vi "Create.vi"(8 "error in (no error)":errorcluster, 10 "Data File":path) -> (0 "error out":errorcluster, 3 "Account Database out":refnum<class "Account Database.lvclass">)   [LabVIEW 2020, in "Account Database.lvclass"]
uses:
  Account Database.lvclass
  Account Database.lvclass/Account Database.ctl
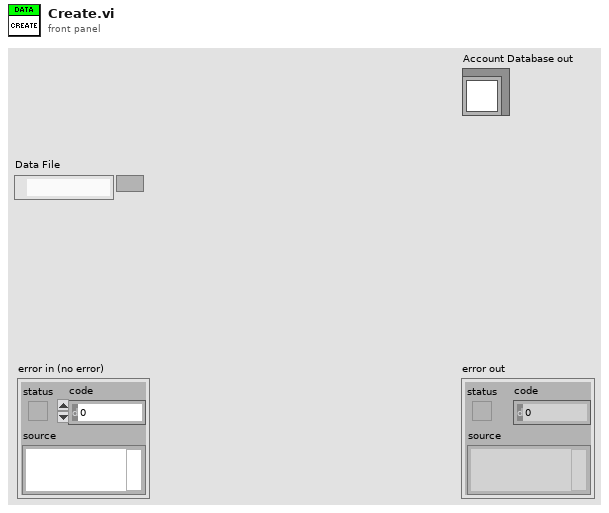
[diagram p1: front panel]
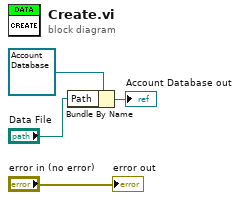
[diagram p0: block diagram]
diagram:
  n1 = Bundle By Name(cluster=refnum<class "Account Database.lvclass"> refnum ("Account Database in"), "Path"="Data File") -> (→"Account Database out":refnum<class "Account Database.lvclass">)
  "error out" <- "error in (no error)"
